vi "test.event_create.vi"   [LabVIEW 2020]
uses:
  990e7071-dbe3-43dc-84d2-0d074c4f9026.vi
  Nominal Client/Nominal Client.lvclass
  <vilib>/numeric/Random Number (Range) DBL.vi
types:
  T1 = cluster{"Properties":map{string, string}, "Labels":string[]}
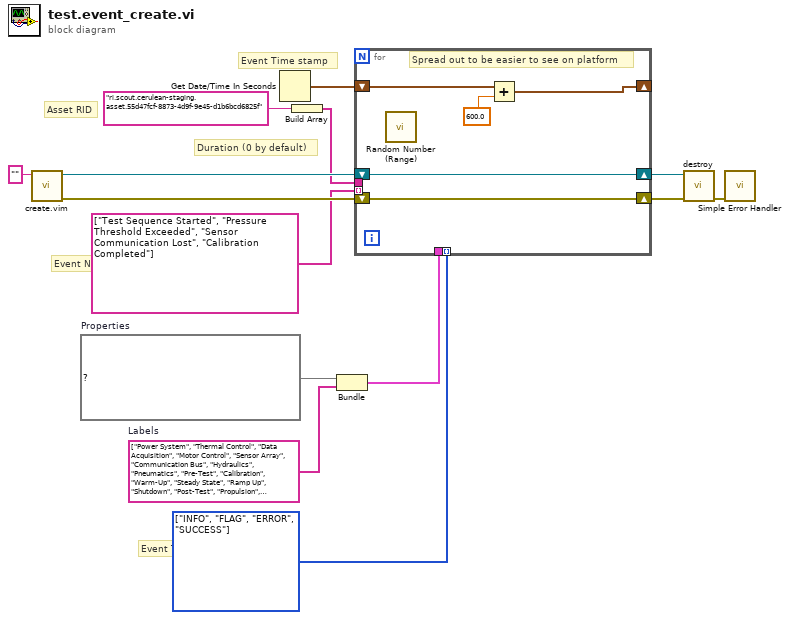
[diagram p0: block diagram]
diagram:
  w2 = string[] ["Power System", "Thermal Control", "Data Acquisition", "Motor Control", "Sensor Array", "Communication Bus", "Hydraulics", "Pneumatics", "Pre-Test", "Calibration", "Warm-Up", "Steady State", "Ramp Up", "Shutdown", "Post-Test", "Propulsion", "Avionics", "Guidance", "Telemetry", "Environmental Control", "Flight Control", "Automated", "Manual Override", "Nominal Operation", "Test Milestone", "Configuration Change", "Operator Action", "System Health", "Critical", "Routine", "Diagnostic", "Maintenance"]  # Labels
  w3 = map{string, string} {"channel"="24.0", "configuration"="Test Stand A", "current"="Baseline", "cycle_count"="Modified", "equipment_id"="100.3", "firmware_version"="1000", "flow_rate"="Config 1", "location"="120", "mode"="240", "operator"="John Smith", "pressure_setpoint"="Test Stand C", "run_number"="12.5", "severity"="v2.0.1", "software_version"="500", "status"="v1.2.3", "subsystem"="fw_3.4.0", "temperature_setpoint"="Test Stand B", "test_id"="25.5", "test_stand"="Jane Doe", "voltage"="Config 2"}  # Properties
  w5 = enum16{"INFO", "FLAG", "ERROR", "SUCCESS"}[] [enum."INFO", enum."FLAG", enum."ERROR", enum."SUCCESS"] items=["INFO", "FLAG", "ERROR", "SUCCESS"] ("type")
  # "Event Time stamp"
  # "Duration (0 by default)"
  # "Event Type"
  # "Event Name"
  # "Asset RID"
  n1 = call "create.vim"("API Token (string or path)"="") -> ("error out"=w8:errorcluster, "Nominal Client"=w9:refnum<class "Nominal Client.lvclass">)  [unwired: 9 in]
  n2 = Get Date/Time In Seconds() -> (seconds since 1Jan1904=w4:timestamp)
  n3 = Build Array("ri.scout.cerulean-staging.asset.55d47fcf-8873-4d9f-9e45-d1b6bcd6825f" ("Asse")) -> (w7:string[])
  n4 = Bundle("Properties"=w3, "Labels"=w2) -> (w1:T1)  [unwired: 1 in]
  n5 = for {
    tunnel: w7 -> [_]
    shift-right: [w16] -> w14
    shift-left: w9 -> [w16]
    shift-right: [w15] -> w13
    shift-left: w8 -> [w15]
    tunnel: w5 -> [_] mode=indexing
    tunnel: string[] ["Test Sequence Started", "Pressure Threshold Exceeded", "Sensor Communication Lost", "Calibration Completed"] ("Name") -> [_] mode=indexing
    shift-right: [w17] -> _
    shift-left: w4 -> [w18]
    tunnel: w1 -> [_]
    # "Spread out to be easier to see on platform"
    n6 = call-poly <vilib>:"Random Number (Range).vi"() -> ()  [unwired: 11 in, 1 out]
    n7 = Add(x=w18, y=600.0) -> (x+y=w17:timestamp)
  }
  n8 = call "destroy.vi"("error in"=w13, "Nominal Client"=w14) -> ("error out"=w11:errorcluster)  [unwired: 9 in]
  n9 = call <vilib>:"Simple Error Handler.vi"("error in (no error)"=w11) -> ()  [unwired: 4 in, 5 out]
